vi "registerObserverEvent.vi"(8 "error in":errorcluster, 11 "ObserverClass in":refnum<class "ObserverClass.lvclass">) -> (0 "error out":errorcluster, 1 "EventReg":refnum<event-registration>, 2 "ObservableName out":string[](array[string]), 3 "ObserverClass out":refnum<class "ObserverClass.lvclass">)   [LabVIEW 2025, in "ObserverClass.lvlib" / "ObserverClass.lvclass"]
doc: "Register Observer Event for each Observable"
uses:
  ObserverClass.lvclass
  ObserverClass.lvclass/ObserverClass.ctl
  Controls/observerControl.ctl
panel:
  out "ObserverEvent out":refnum<user-event>[](array[refnum])
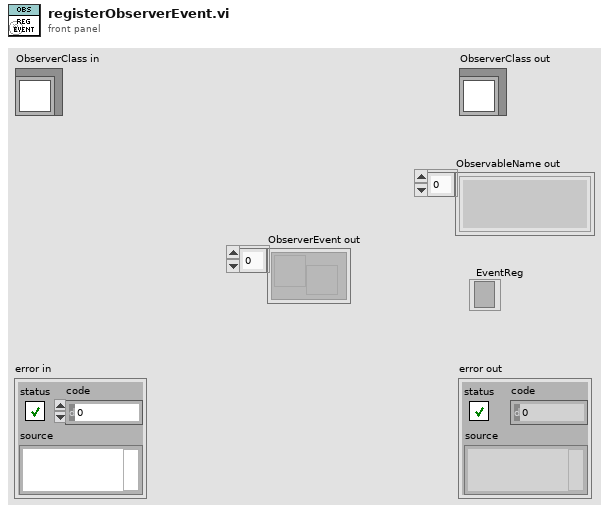
[diagram p1: front panel]
types:
  T1 = map{string, cluster{"ObserverEvent":refnum<user-event>, "ObserverNr":u64, "ObservableValue":variant}}
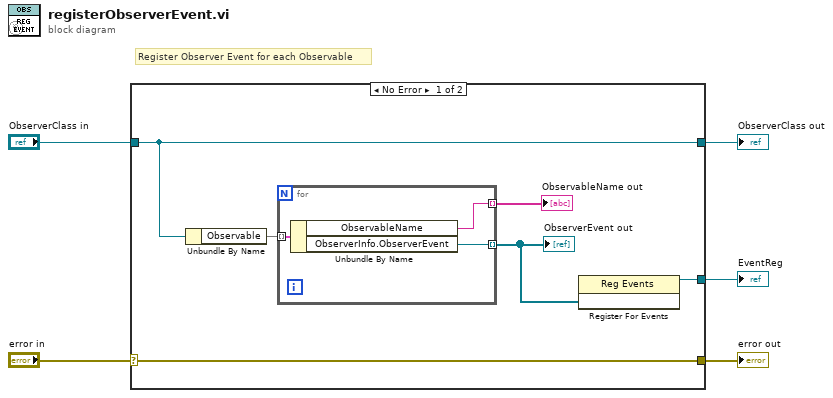
[diagram p0: block diagram]
diagram:
  # "Register Observer Event for each Observable"
  n1 = case shown="No Error" "error in" {
    selector: "error in" -> [w11 w16]
    tunnel: [w11 w16] -> w4
    tunnel: [w10 w15] -> w2
    tunnel: "ObserverClass in" -> [w10 w15]
    tunnel: [w6 _] -> w1
    frame No Error {
      n2 = Unbundle By Name(w10) -> ("Observable"=w9:T1)
      n3 = for {
        tunnel: w9 -> [w14] mode=indexing
        tunnel: [w13] -> w8 mode=indexing
        tunnel: [w12] -> w7 mode=indexing
        n4 = Unbundle By Name(w14) -> ("ObservableName"=w13:string, "ObserverInfo.ObserverEvent"=w12:refnum<user-event>)
      }
      "ObservableName out" <- w8
      "ObserverEvent out" <- w7
      n5 = register-events(w7) -> (reference out=w6:refnum<event-registration>)  [unwired: 2 in, 1 out]
    }
    frame Error {
    }
  }
  "error out" <- w4
  "ObserverClass out" <- w2
  "EventReg" <- w1
